vi "tank_auto_sub.vi"(8 "logging in":i32[](array[numeric]), 9 "Target Heading (Degrees)":i16, 10 "Drive Control":T2={"Left X"=0, "Left Y"=0, "Right Y"=0, "Power (100)"=100, "Wait (ms)"=100, "Enc/Deg Target"=0, "Move Type"=enum."Wait"} {"Power (100)" min=-100 max=100}, 11 "NXT/EV3":T1) -> (0 "logging out":i32[](array[numeric]), 3 "NXT/EV3 out":T1)   [LabVIEW 2012, in "Serenity_mk2.lvrbt"]
uses:
  Serenity_mk2.lvrbt
  SubVIs/auto_drive_TYP.ctl
  <vilib>/NXT/Subs/LVHSConnector.ctl
  <vilib>/NXT/LegoClasses/BrickReference/BrickReference.lvclass
  <vilib>/FTC/FTC ControllerState.ctl
  <vilib>/FTC/FTC POVState.ctl
  <vilib>/NXT/Hardware/Plugins/Tetrix DC Motor/TetrixDCMotorAddress.ctl
  <vilib>/NXT/HiTechnic/HiTechnic Controls/HiTechnic Port.ctl
  <vilib>/NXT/Block Support/NXT_InputPort.ctl
  <vilib>/FTC/FTC Calculate Drive Power - Tank.vi
  <vilib>/NXT/NXTIO Xnodes/NXTIONodeSubVIs/TETRIX IO Move DC Motors.vi
  <vilib>/NXT/Dual Mode Library/Waits/Wait_Num(msec).vi
  <vilib>/NXT/NXTIO Xnodes/NXTIONodeSubVIs/TETRIX IO Motor Status.vi
  <vilib>/NXT/Dual Mode Library/Display/drawNumber.vi
  <vilib>/NXT/NXTIO Xnodes/AddressXNode/NXTIOAddress.xnode
  <vilib>/NXT/NXTIO Xnodes/NXTIOXNode/NXTIO.xnode
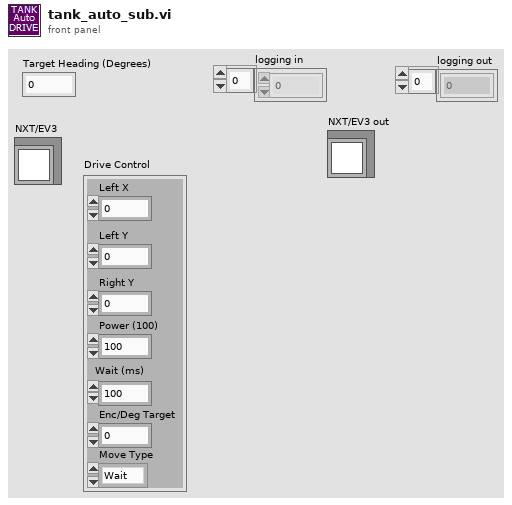
[diagram p1: front panel]
types:
  T1 = typedef "LVHSConnector.ctl" = refnum<class "BrickReference.lvclass">
  T2 = typedef "auto_drive_TYP.ctl" = cluster{"Left X":i8, "Left Y":i8, "Right Y":i8, "Power (100)":i8, "Wait (ms)":u32, "Enc/Deg Target":i32, "Move Type":enum16{"Relative Degrees", "Wait", "Encoder"}}
  T3 = typedef "FTC ControllerState.ctl" = cluster{"Left X":i8, "Left Y":i8, "Right X":i8, "Right Y":i8, "Button Encoding 9-12":u8, "Button Encoding 1-8":u8, "POV":T4}
  T4 = typedef "FTC POVState.ctl" = i8
  T5 = typedef "TetrixDCMotorAddress.ctl" = i32
  T6 = typedef "HiTechnic Port.ctl" = cluster{"Port":T7, "MUX Port":u8}
  T7 = typedef "NXT_InputPort.ctl" = u32
  T8 = cluster{"TetrixDCMotor":T5, "TetrixDCMotor 2":T5}
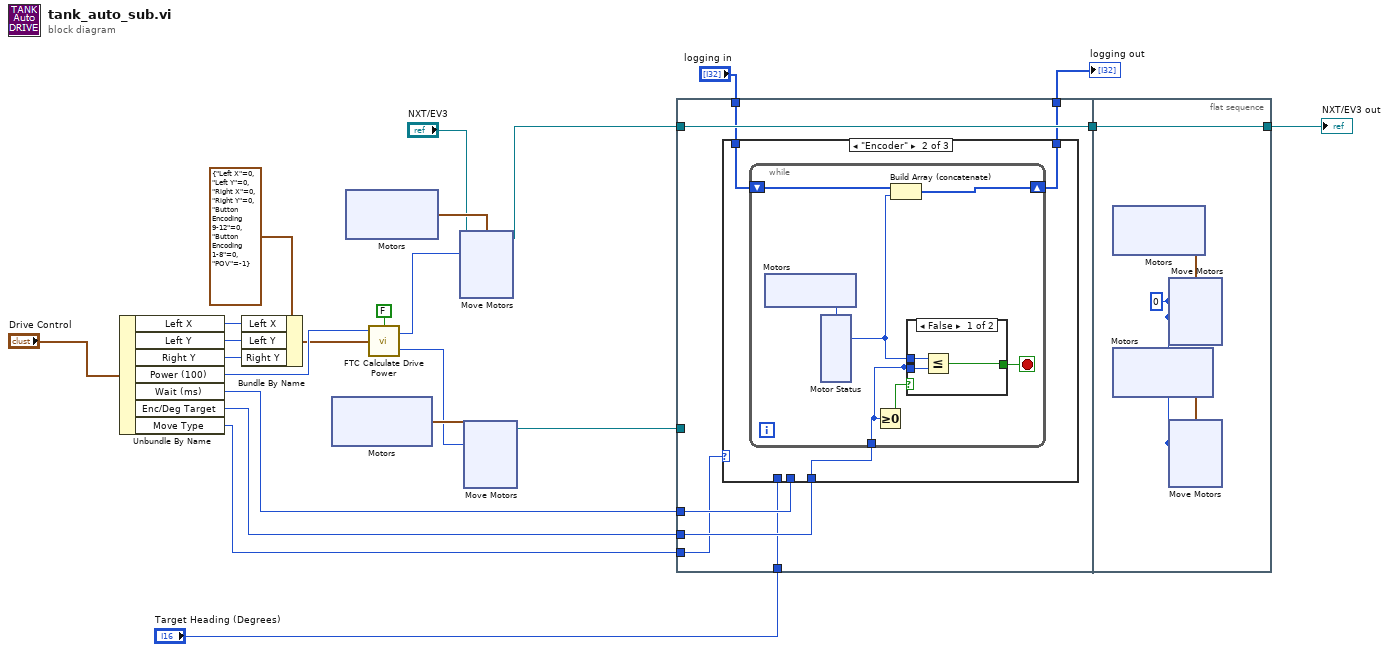
[diagram p0: block diagram]
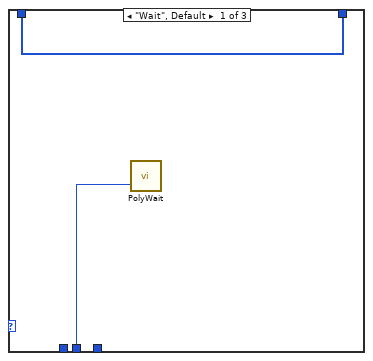
[diagram p2: hidden frame]
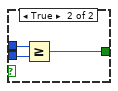
[diagram p3: hidden frame]
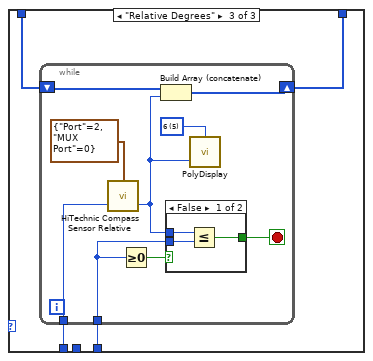
[diagram p4: hidden frame]
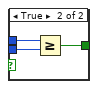
[diagram p5: hidden frame]
diagram:
  n1 = Unbundle By Name("Drive Control") -> ("Left X"=w17:i8, "Left Y"=w16:i8, "Right Y"=w15:i8, "Power (100)"=w2:i8, "Wait (ms)"=w12:u32, "Enc/Deg Target"=w10:i32, "Move Type"=w9:enum16{"Relative Degrees", "Wait", "Encoder"})
  n2 = Bundle By Name(cluster=T3 {"Left X"=0, "Left Y"=0, "Right X"=0, "Right Y"=0, "Button Encoding 9-12"=0, "Button Encoding 1-8"=0, "POV"=-1} ("Controller State"), "Left X"=w17, "Left Y"=w16, "Right Y"=w15) -> (w1:T3)
  n3 = xnode ("Motors")() -> ("Motor"=w22:cluster{"TetrixDCMotor":T5, "TetrixDCMotor":T5})
  n4 = xnode ("Motors")() -> ("Motor"=w21:cluster{"TetrixDCMotor":T5, "TetrixDCMotor":T5})
  n5 = call-poly <vilib>:"FTC Calculate Drive Power.vi"("Reverse"=FALSE, "Controller State"=w1, "Power Level (50)"=w2) -> ("Right Motor Power"=w4:i8, "Left Motor Power"=w3:i8)  [unwired: 1 in]
  n6 = xnode ("Move Motors")("Power/Speed 1"=w3, "Motors"=w21, "NXT/EV3"="NXT/EV3") -> ("NXT/EV3"=w14:T1)  [unwired: 1 in]
  n7 = xnode ("Move Motors")("Power/Speed 1"=w4, "Motors"=w22) -> ("NXT/EV3"=w13:T1)  [unwired: 2 in]
  n8 = flat-sequence {
    tunnel: w14 -> [w30]
    tunnel: w13 -> [_]
    tunnel: w12 -> [w29]
    tunnel: [w30] -> w23
    tunnel: w10 -> [w28]
    tunnel: w9 -> [w27]
    tunnel: "Target Heading (Degrees)" -> [w26]
    tunnel: "logging in" -> [w25]
    tunnel: [w24] -> w6
    tunnel: [w80] -> w11
    tunnel: w23 -> [w80]
    frame #0 {
      n9 = case shown="\"Encoder\"" w27 {
        tunnel: w29 -> [w32 _ _]
        tunnel: w28 -> [_ w35 w60]
        tunnel: w26 -> [_ _ w61]
        tunnel: w25 -> [w31 w34 w59]
        tunnel: [w31 w33 w58] -> w24
        frame "Wait", Default {
          n10 = call-poly <vilib>:"PolyWait.vi"("Time (100 msec)"=w32) -> ()  [unwired: 3 in, 1 out]
        }
        frame "Encoder" {
          n11 = while {
            tunnel: w35 -> [w36]
            shift-right: [w41] -> w33
            shift-left: w34 -> [w40]
            stop <- w37 stop-if-true
            n12 = xnode "Motors"() -> ("Motor"=w42:T5)
            n13 = xnode "Motor Status"("Motors"=w42) -> ("Position 1"=w38:i32)  [unwired: 1 in, 2 out]
            n14 = Greater Or Equal To 0?(x=w36) -> (x >= 0?=w39:bool)
            n15 = Build Array (concatenate)(w40, w38) -> (w41:i32[])
            n16 = case shown="False" w39 {
              tunnel: w36 -> [_ w47]
              tunnel: w38 -> [w45 w48]
              tunnel: [w43 w46] -> w37
              tunnel: w36 -> [w44 _]
              frame False {
                n17 = Less Or Equal?(x=w45, y=w44) -> (x <= y?=w43:bool)
              }
              frame True {
                n18 = Greater Or Equal?(x=w48, y=w47) -> (x >= y?=w46:bool)
              }
            }
          }
        }
        frame "Relative Degrees" {
          n19 = while {
            tunnel: w61 -> [w69]
            tunnel: w60 -> [w66]
            shift-right: [w64] -> w58
            shift-left: w59 -> [w62]
            stop <- w68 stop-if-true
            w67 = i16 5 items=["1", "2", "3", "4", "5", "6", "7", "8", "9", "10", "11", "12"] ("Line")
            n20 = call <vilib>:"HiTechnic Compass Sensor Relative.vi"("Target Heading (Degrees)"=w69, "Port/MUX"=T6 {"Port"=2, "MUX Port"=0}) -> ("Relative Heading (Degrees)"=w63:i32)  [unwired: 1 in, 1 out]
            n21 = Greater Or Equal To 0?(x=w66) -> (x >= 0?=w65:bool)
            n22 = Build Array (concatenate)(w62, w63) -> (w64:i32[])
            n23 = case shown="False" w65 {
              tunnel: w66 -> [w71 w76]
              tunnel: [w73 w75] -> w68
              tunnel: w63 -> [w72 w74]
              frame False {
                n24 = Less Or Equal?(x=w72, y=w71) -> (x <= y?=w73:bool)
              }
              frame True {
                n25 = Greater Or Equal?(x=w74, y=w76) -> (x >= y?=w75:bool)
              }
            }
            n26 = call-poly <vilib>:"PolyDisplay.vi"("number"=w63, "Line"=w67) -> ()  [unwired: 2 in, 1 out]
          }
        }
      }
    }
    frame #1 {
      w77 = i8 0 ("Power/Speed 1")
      n27 = xnode "Motors"() -> ("Motor"=w79:cluster{"TetrixDCMotor":T5, "TetrixDCMotor":T5})
      n28 = xnode "Motors"() -> ("Motor"=w78:cluster{"TetrixDCMotor":T5, "TetrixDCMotor":T5})
      n29 = xnode "Move Motors"("Power/Speed 2"=w77, "Power/Speed 1"=w77, "Motors"=w79) -> ()  [unwired: 1 in, 1 out]
      n30 = xnode "Move Motors"("Power/Speed 2"=w77, "Power/Speed 1"=w77, "Motors"=w78) -> ()  [unwired: 1 in, 1 out]
    }
  }
  "NXT/EV3 out" <- w11
  "logging out" <- w6
